vi "Publish Message to Email Subscription.vi"() -> ()   [LabVIEW 2015]
doc: "Demonstrates how to publish a message to an existing subscription to an SNS topic."
uses:
  Core/HTTP Request/Region.ctl
  Core/HTTP Request/AWS Credentials.ctl
  Core/HTTP Request/HTTP Request.lvclass
  SNS/Topic/Topic.lvclass
  SNS/Subscription/Subscription.lvclass
panel:
  in  "Email Body":string
  in  "Email Subject":string
  in  "Region":T1
  in  "Secret Key":string
  in  "Access Key":string
  in  "Topic Name":string
  # "Overview: Demonstrates how to publish a message to an existing subscription to an SNS topic.\nRequirements: NI Cloud Toolkit for AWS and a registered Amazon AWS account\nInstructions:\n1. Make sure you have already run the Create SNS Topic and Email Subscription.vi example, and that you have clicked the Confirm subscription link in the confirmation email you received.\n2. Specify the Access Key and Secret Key for your AWS account. You can create an account at http://aws.amazon.com.\n3. Specify the same Topic Name you used in the Create SNS Topic and Email Subscription.vi example.\n4. Specify an Email Subject and Email Body for the email to be sent.\n5. Run the VI. The specified SNS Topic will publish a message to subscribed email address."
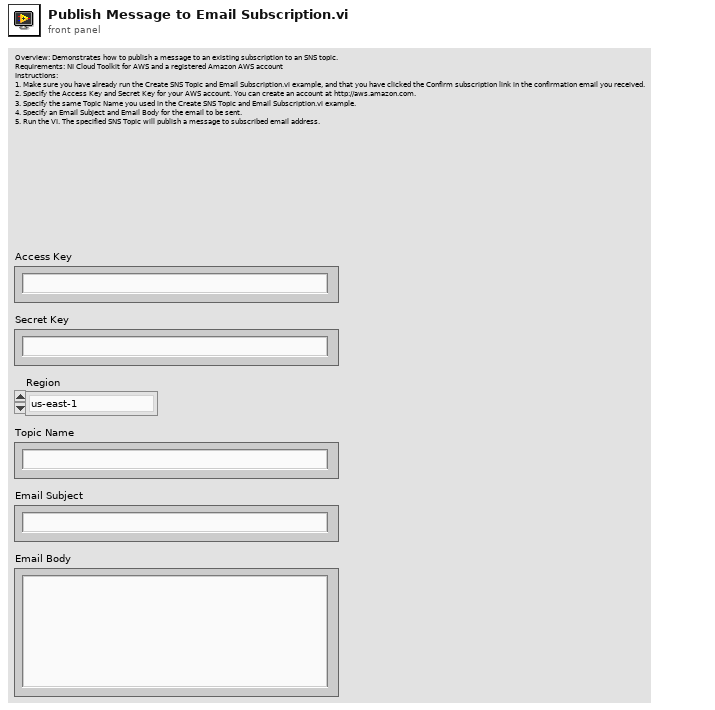
[diagram p1: front panel]
types:
  T1 = typedef "NI_AWS_Core.lvlib/HTTP Request.lvclass/Region.ctl" = enum16{"us-east-1", "us-east-2", "us-west-1", "us-west-2", "ap-northeast-1", "ap-northeast-2", "ap-southeast-1", "ap-southeast-2", "ca-central-1", "eu-central-1", "eu-west-1", "eu-west-2", "sa-east-1"}
  T2 = typedef "NI_AWS_Core.lvlib/HTTP Request.lvclass/AWS Credentials.ctl" = cluster{"Access Key":string, "Secret Key":string}
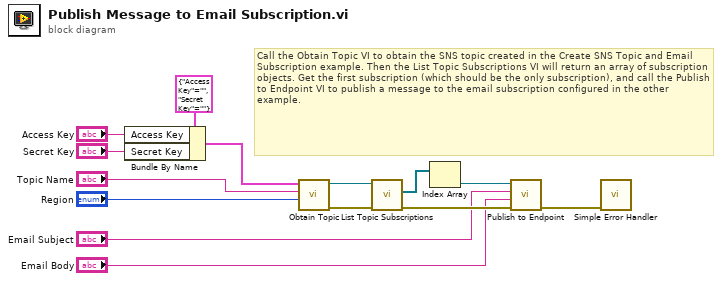
[diagram p0: block diagram]
diagram:
  # "Call the Obtain Topic VI to obtain the SNS topic created in the Create SNS Topic and Email Subscription example. Then the List Topic Subscriptions VI will return an array of subscription objects. Get the first subscription (which should be the only subscription), and call the Publish to Endpoint VI to publish a message to the email subscription configured in the other example."
  n1 = Bundle By Name(cluster=T2 {"Access Key"="", "Secret Key"=""} ("AWS Credentials"), "Access Key"="Access Key", "Secret Key"="Secret Key") -> (w11:T2)
  n2 = call "Obtain Topic.vi"("Region"="Region", "Name"="Topic Name", "AWS Credentials"=w11) -> ("error out"=w8:errorcluster, "Topic out"=w6:refnum<class "Topic.lvclass">)  [unwired: 7 in]
  n3 = call "List Topic Subscriptions.vi"("error in (no error)"=w8, "Topic in"=w6) -> ("error out"=w7:errorcluster, "Subscriptions"=w5:refnum<class "Subscription.lvclass">[])  [unwired: 7 in, 1 out]
  n4 = Index Array(array=w5) -> (element=w3:refnum<class "Subscription.lvclass">)  [unwired: 1 in]
  n5 = call "Publish to Endpoint.vi"("error in (no error)"=w7, "Message"="Email Body", "Subject"="Email Subject", "Subscription in"=w3) -> ("error out"=w4:errorcluster)  [unwired: 6 in, 1 out]
  n6 = call <vilib>:"Simple Error Handler.vi"("error in (no error)"=w4) -> ()  [unwired: 4 in, 5 out]
